vi "CmdConsole.Run.vi"(8 "error in (no error)":errorcluster, 10 "StdOutQ":string, 11 "CmdConsole in":refnum<class "CmdConsole.lvclass">) -> (0 "error out":errorcluster, 2 "Running":bool, 3 "CmdConsole out":refnum<class "CmdConsole.lvclass">)   [LabVIEW 2024, in "CmdConsole.lvclass"]
uses:
  CmdConsole.lvclass
  CmdConsole.lvclass/CmdConsole.ctl
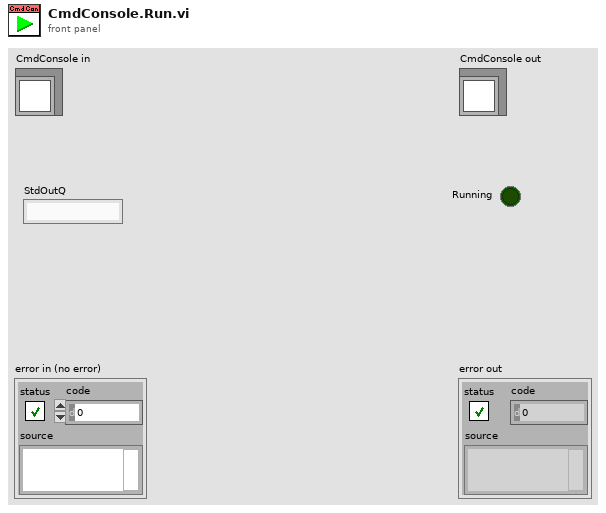
[diagram p1: front panel]
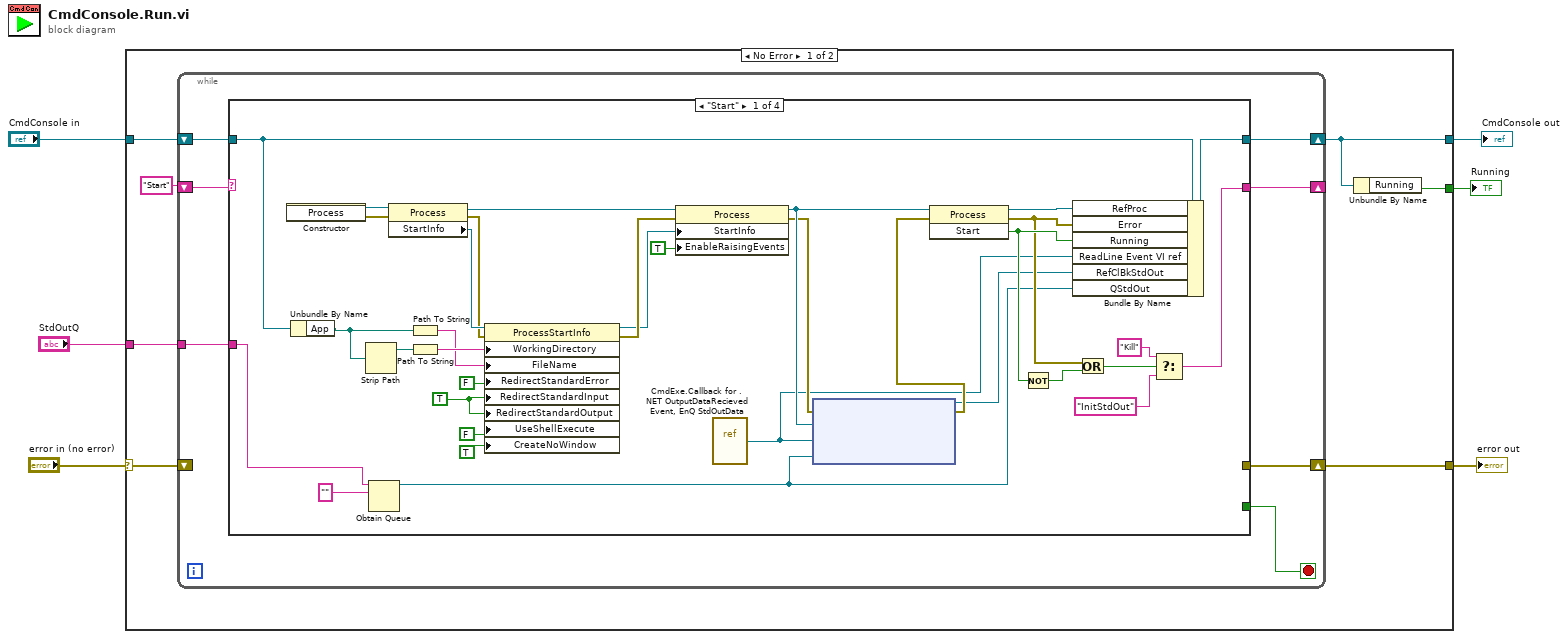
[diagram p0: block diagram]
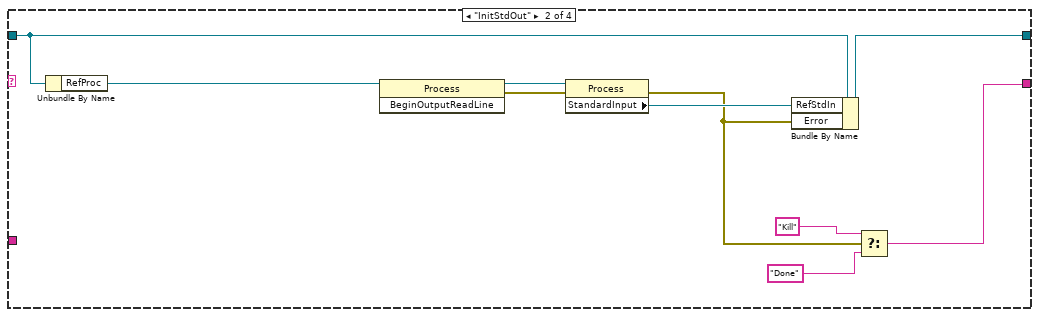
[diagram p2: hidden frame]
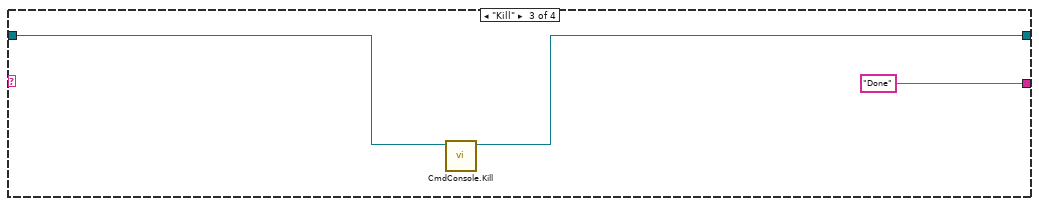
[diagram p3: hidden frame]
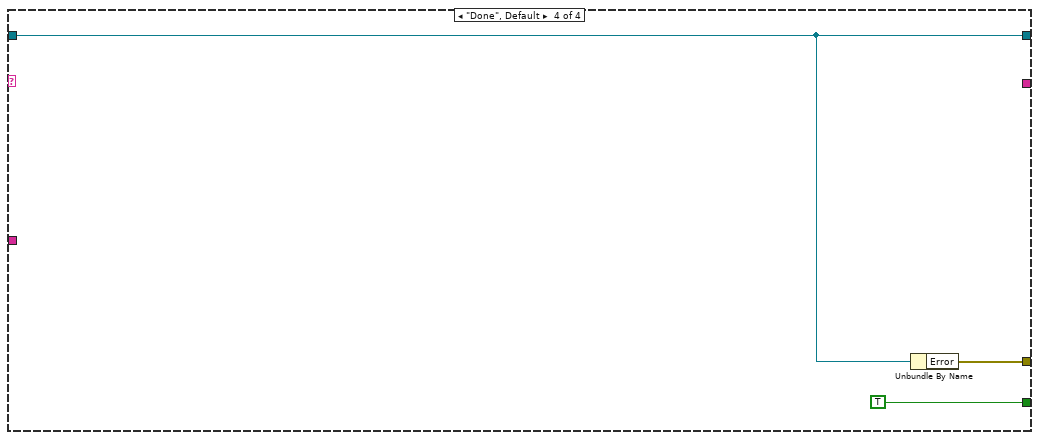
[diagram p4: hidden frame]
diagram:
  n1 = case shown="No Error" "error in (no error)" {
    selector: "error in (no error)" -> [w10 w72]
    tunnel: [w11 w72] -> w5
    tunnel: [w9 w71] -> w3
    tunnel: "CmdConsole in" -> [w13 w71]
    tunnel: [w8 _] -> w2
    tunnel: "StdOutQ" -> [w7 _]
    frame No Error {
      n2 = while {
        shift-right: [w19] -> w9
        shift-left: w13 -> [w20]
        shift-right: [w17] -> _
        shift-left: "Start" -> [w18]
        shift-right: [w15] -> w11
        shift-left: w10 -> [_]
        tunnel: w7 -> [w14]
        stop <- w16 stop-if-true
        n3 = case shown="\"Start\"" w18 {
          tunnel: w20 -> [w54 w64 w65 w69]
          tunnel: [w39 w62 w66 w69] -> w19
          tunnel: [w31 w59 "Done" _] -> w17
          tunnel: [_ _ _ TRUE] -> w16
          tunnel: [_ _ _ w68] -> w15
          tunnel: w14 -> [w28 _ _ _]
          frame "Start" {
            w40 = TRUE ("UseShellExecute")
            n4 = constructor class="Process"() -> (reference out=w53:refnum<k24>, error out=w52:errorcluster)  [unwired: 3 in, 1 out]
            n5 = Unbundle By Name(w54) -> ("App"=w41:path)
            n6 = Strip Path(path=w41) -> (stripped path=w44:path)  [unwired: 1 out]
            n7 = Obtain Queue(name (unnamed)=w28, element data type="") -> (queue out=w22:refnum<queue>)  [unwired: 3 in, 2 out]
            n8 = property class="Process"(reference=w53, error in=w52) -> (reference out=w45:refnum<k24>, error out=w46:errorcluster, "StartInfo"=w51:refnum<k24>)
            n9 = Path To String(path=w41) -> (string=w42:string)
            n10 = Path To String(path=w44) -> (string=w43:string)
            n11 = property class="ProcessStartInfo"(reference=w51, error in=w46, "WorkingDirectory"=w43, "FileName"=w42, "RedirectStandardError"=FALSE ("UseShellExecute"), "RedirectStandardInput"=w40, "RedirectStandardOutput"=w40, "UseShellExecute"=FALSE, "CreateNoWindow"=TRUE) -> (reference out=w47:refnum<k24>, error out=w48:errorcluster)
            n12 = property class="Process"(reference=w45, error in=w48, "StartInfo"=w47, "EnableRaisingEvents"=TRUE) -> (reference out=w27:refnum<k24>, error out=w25:errorcluster)
            n13 = vi-ref "CmdExe.Callback for .NET OutputDataRecieved Event, EnQ StdOutData.vi"() -> ("vi reference"=w23:refnum<vi>)
            n14 = node(w25, w27, w23, w22) -> (w24:refnum<k27>, w26:errorcluster)  [unwired: 1 in]
            n15 = invoke class="Process" method="Start"(reference=w27, error in=w26) -> (reference out=w38:refnum<k24>, error out=w35:errorcluster, "Start"=w37:bool)  [unwired: 1 in]
            n16 = Not(x=w37) -> (.not. x?=w36:bool)
            n17 = Bundle By Name(cluster=w54, "RefProc"=w38, "Error"=w35, "Running"=w37, "ReadLine Event VI ref"=w23, "RefClBkStdOut"=w24, "QStdOut"=w22) -> (w39:refnum<class "CmdConsole.lvclass">)
            n18 = Or(x=w35, y=w36) -> (x .or. y?=w34:bool)
            n19 = Select(t="Kill", s=w34, f="InitStdOut") -> (s? t:f=w31:string)
          }
          frame "InitStdOut" {
            n20 = Unbundle By Name(w64) -> ("RefProc"=w56:refnum<k24>)
            n21 = invoke class="Process" method="BeginOutputReadLine"(reference=w56) -> (reference out=w57:refnum<k24>, error out=w58:errorcluster)  [unwired: 2 in, 1 out]
            n22 = property class="Process"(reference=w57, error in=w58) -> (error out=w55:errorcluster, "StandardInput"=w63:refnum<k24>)  [unwired: 1 out]
            n23 = Bundle By Name(cluster=w64, "RefStdIn"=w63, "Error"=w55) -> (w62:refnum<class "CmdConsole.lvclass">)
            n24 = Select(t="Kill", s=w55, f="Done") -> (s? t:f=w59:string)
          }
          frame "Kill" {
            n25 = call "CmdConsole.Kill.vi"("CmdConsole in"=w65) -> ("CmdConsole out"=w66:refnum<class "CmdConsole.lvclass">)  [unwired: 9 in, 1 out]
          }
          frame "Done", Default {
            n26 = Unbundle By Name(w69) -> ("Error"=w68:errorcluster)
          }
        }
      }
      n27 = Unbundle By Name(w9) -> ("Running"=w8:bool)
    }
    frame Error {
    }
  }
  "error out" <- w5
  "CmdConsole out" <- w3
  "Running" <- w2
